vi "SetCursorPos(x,y).vi"(0 "vi reference":refnum<vi>, 7 "(X,Y)":T1, 11 "Error in":errorcluster) -> (4 "Sucess?":i32, 15 "Error out":errorcluster)   [LabVIEW 2013]
doc: "This VI moves the mouse pointer to the desired position. \nInputs:\n1.VI path: The VI inside which the pointer has to be moved\n2.(X,Y): The co-ordinates of the desired position with respect to origin on the Front Panel\n3.Front Panel Window:Open: Used to indicate whether the VI's Front Panel has to be opened before moving the mouse pointer\n4.Error in\n\nOutputs:\n1.Success: Returns a non-zero number(1) to indicate the move has happened and returns 0 to indicate that the move din't happen.\n2.Error out"
uses:
  <vilib>/Utility/miscctls.llb/LVPointTypeDef.ctl
  <vilib>/Utility/miscctls.llb/LVPositionTypeDef.ctl
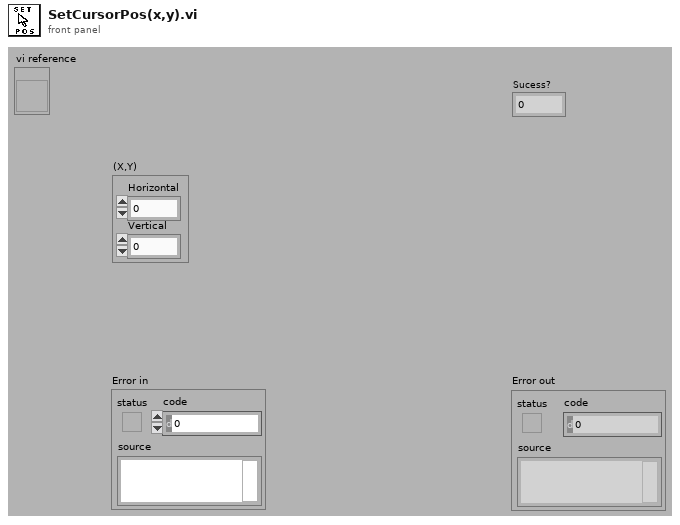
[diagram p1: front panel]
types:
  T1 = typedef "LVPointTypeDef.ctl" = cluster{"Horizontal":i16, "Vertical":i16}
  T2 = typedef "LVPositionTypeDef.ctl" = cluster{"Left":i32, "Top":i32}
  T3 = typedef "LVRectTypeDef.ctl" = cluster{"Left":i16, "Top":i16, "Right":i16, "Bottom":i16}
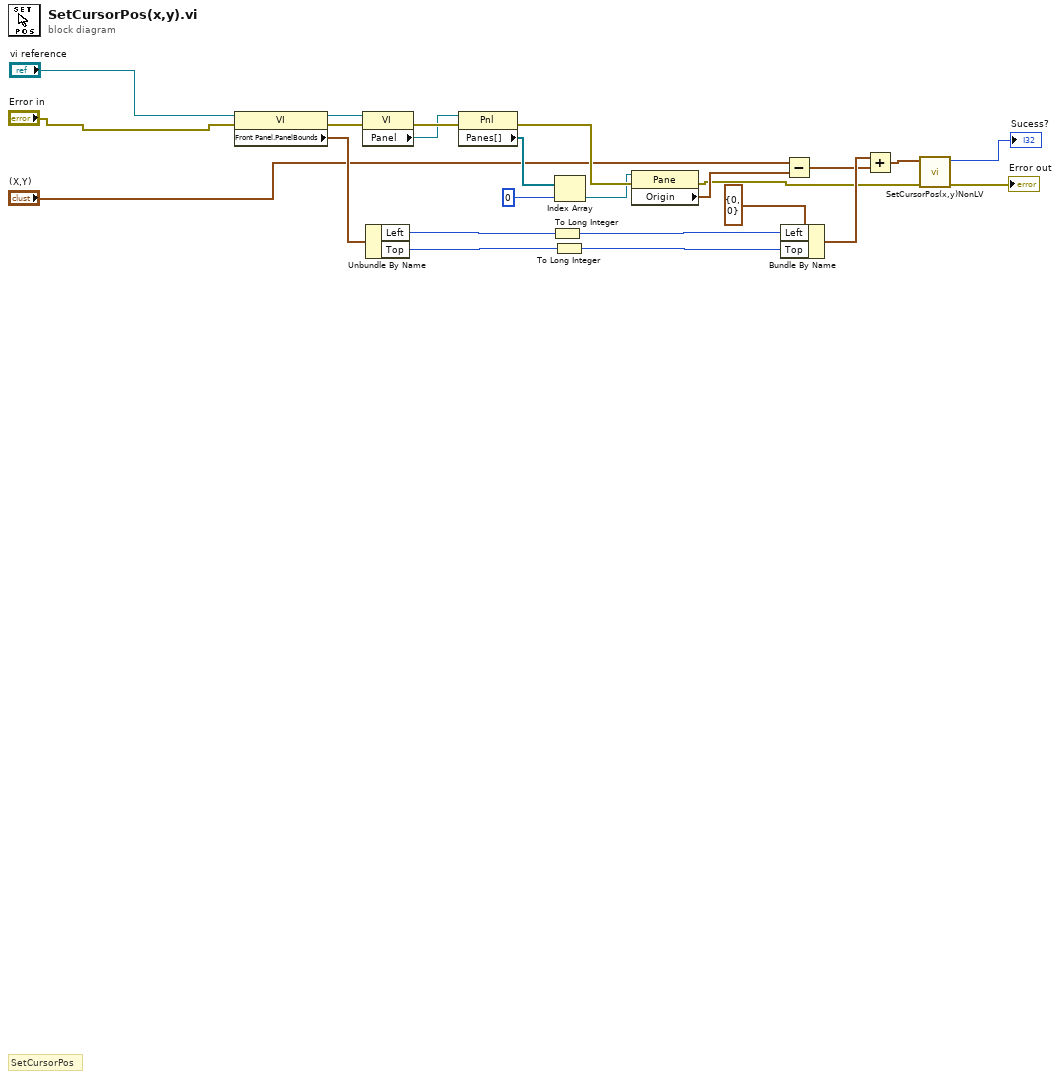
[diagram p0: block diagram]
diagram:
  # "SetCursorPos"
  n1 = property class="VI"(reference="vi reference", error in="Error in") -> (reference out=w18:refnum<vi>, error out=w19:errorcluster, "Front Panel.PanelBounds"=w17:T3)
  n2 = property class="VI"(reference=w18, error in=w19) -> (error out=w20:errorcluster, "Panel"=w6:refnum<vi>)  [unwired: 1 out]
  n3 = Unbundle By Name(w17) -> ("Left"=w14:i16, "Top"=w11:i16)
  n4 = property class="Pnl"(reference=w6, error in=w20) -> (error out=w24:errorcluster, "Panes[]"=w21:refnum<vi>[])  [unwired: 1 out]
  n5 = To Long Integer(number=w14) -> (32bit integer=w13:i32)
  n6 = To Long Integer(number=w11) -> (32bit integer=w12:i32)
  n7 = Index Array(array=w21, index=0) -> (element=w23:refnum<vi>)
  n8 = property class="Pane"(reference=w23, error in=w24) -> (error out=w3:errorcluster, "Origin"=w9:T1)  [unwired: 1 out]
  n9 = Bundle By Name(cluster=T2 {"Left"=0, "Top"=0} ("Position"), "Left"=w13, "Top"=w12) -> (w16:T2)
  n10 = Subtract(x="(X,Y)", y=w9) -> (x-y=w15:T1)
  n11 = Add(x=w16, y=w15) -> (x+y=w4:T2)
  n12 = call "SetCursorPos(x,y)NonLV.vi"("error in"=w3, "RelativePosition"=w4) -> ("error out"=→"Error out":errorcluster, "sucess"=→"Sucess?":i32)  [unwired: 8 in]
